vi "Bus Interface.vi"(0 "AddressSpace":refnum<class "AddressSpace.lvclass">, 1 "abort":bool, 5 "instruction":T2, 9 "input valid":bool) -> (6 "response":T1, 10 "done":bool, 14 "ready for input":bool)   [LabVIEW 2017, in "BuckBoost.lvlib" / "AddressSpace.lvclass"]
uses:
  AddressSpace.lvclass
  <instrlib>/_niInstr/Instruction Framework/v1/FPGA/Interfaces/Address Space/Address Space Instruction.ctl
  <instrlib>/_niInstr/Instruction Framework/v1/FPGA/Typedefs/Response.ctl
  AddressSpace.lvclass/AddressSpace.ctl
  <vilib>/Utility/error.llb/Clear Errors.vi
  <vilib>/rvi/Emulation/niFpgaSctlEmulationGetInTimedLoop.vi
  <vilib>/rvi/DataTransferAndStorage/Container/Common/niFpgaContainerExecOnDevCompGetState.vi
  <vilib>/rvi/Emulation/niFpgaEmulationIsFPGAContextNoSignature.vi
  <vilib>/rvi/DataTransferAndStorage/Container/Common/niFpgaContainerGetUniqueNameForEmu.vi
  <vilib>/rvi/Memory/Memory_Emulation/niFpgaMemoryEmulationCacheClearOnFirstRun.vi
  <vilib>/rvi/Memory/Memory_Emulation/nirvimemoryEmulationManagerCache_MakeExclusive.vi
  <vilib>/rvi/Memory/Memory_Emulation/niFpgaMemoryEmulationValidateCache.vi
  <vilib>/rvi/Memory/Memory_Emulation/nirvimemoryEmulationManagerCache_InsertValue.vi
  <vilib>/rvi/Memory/Memory_Emulation/nirvimemoryEmulationManagerCache_ReleaseExclusive.vi
  <vilib>/rvi/Memory/Memory_Emulation/nirvimemoryEmulationManagerCache_GetValue.vi
  <vilib>/rvi/Memory/Memory_Emulation/nirvimemoryEmulationManagerCache_SetValue.vi
  <vilib>/rvi/Emulation/niFpgaProcessEmulError.vi
  <vilib>/rvi/DataTransferAndStorage/Container/XNode/niFpgaContainer.xnode
  <vilib>/rvi/DataTransferAndStorage/Register/Emulation/niFpgaRegisterEmulationRefIn.vi
  <instrlib>/_niInstr/Instruction Framework/v1/FPGA/Typedefs/niInstr Instruction Framework v1 FPGA.lvlib
  <instrlib>/_niInstr/Instruction Framework/v1/FPGA/Interfaces/Address Space/Address Space.lvclass
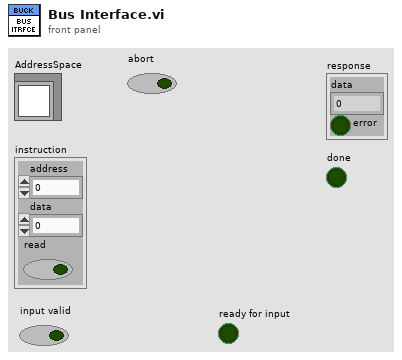
[diagram p1: front panel]
types:
  T1 = typedef "niInstr Instruction Framework v1 FPGA.lvlib/Response.ctl" = cluster{"data":u64, "error":bool}
  T2 = typedef "niInstr Instruction Framework Interfaces v1 FPGA.lvlib/Address Space.lvclass/Address Space Instruction.ctl" = cluster{"address":u32, "data":u64, "read":bool}
  T3 = cluster{"proportional gain":sgl, "integral gain":sgl}
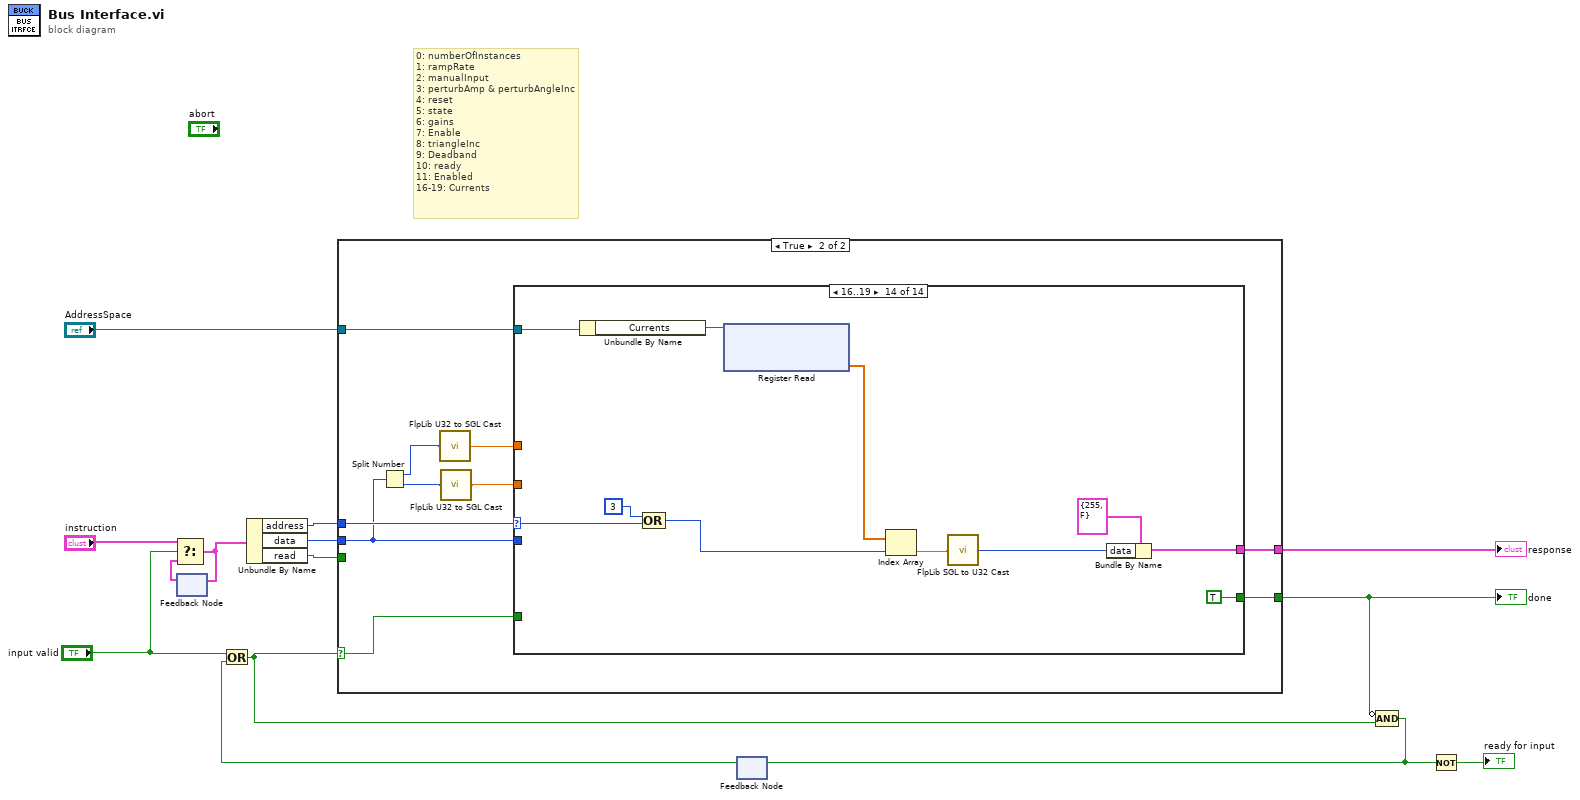
[diagram p0: block diagram]
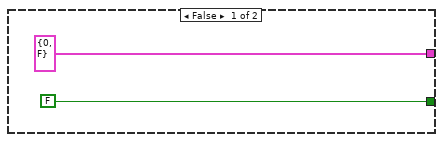
[diagram p2: hidden frame]
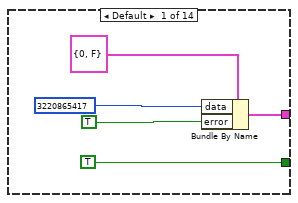
[diagram p3: hidden frame]
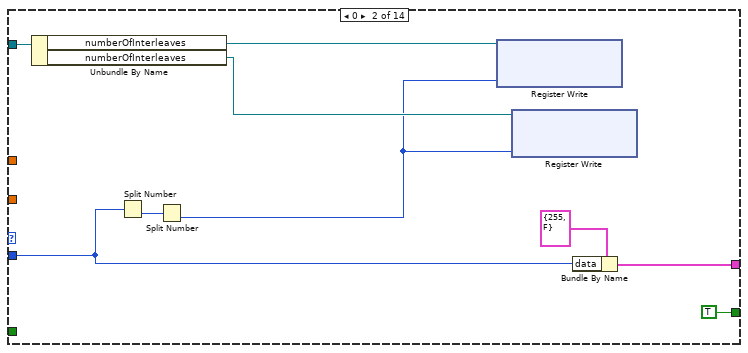
[diagram p4: hidden frame]
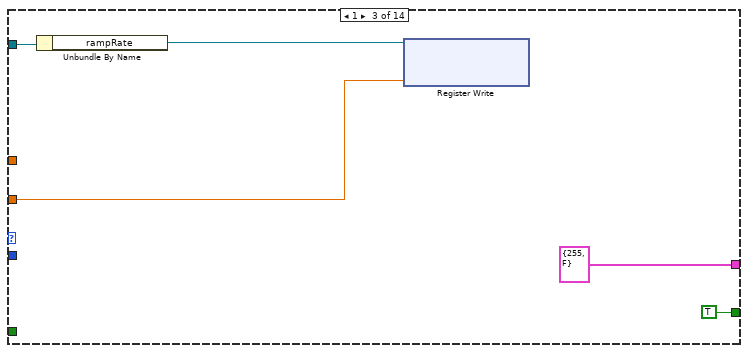
[diagram p5: hidden frame]
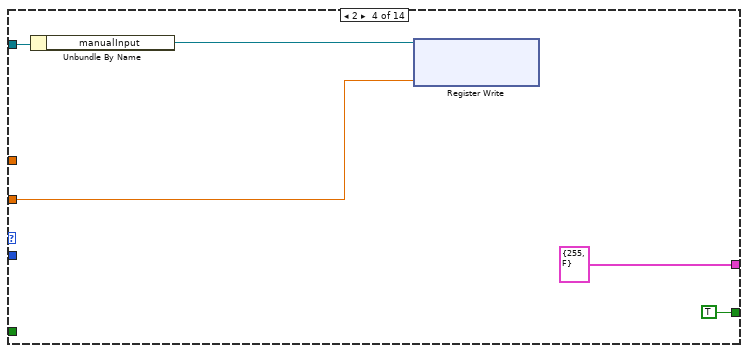
[diagram p6: hidden frame]
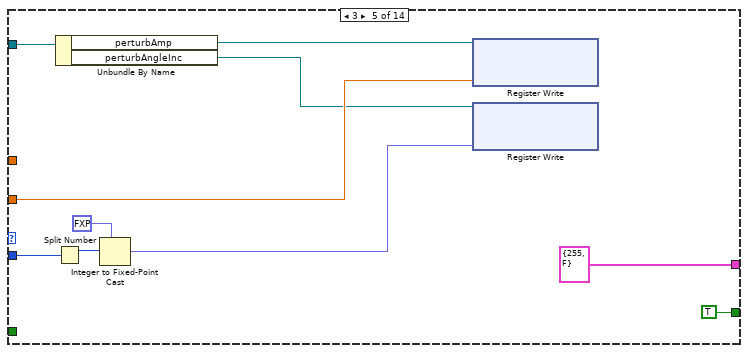
[diagram p7: hidden frame]
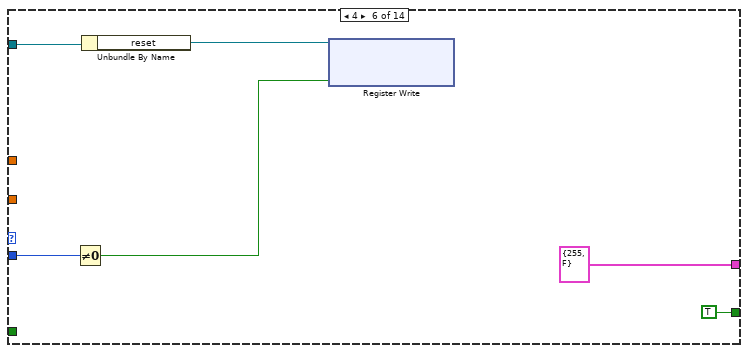
[diagram p8: hidden frame]
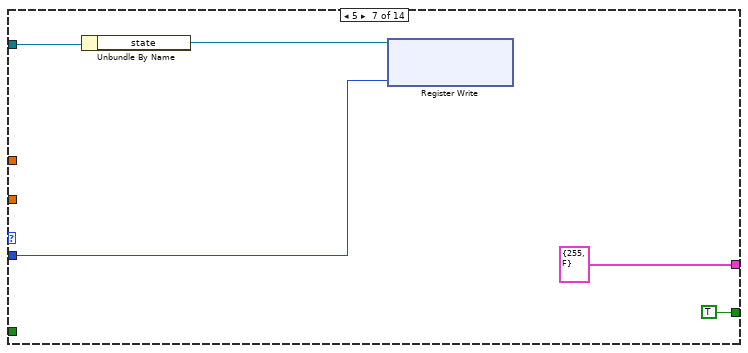
[diagram p9: hidden frame]
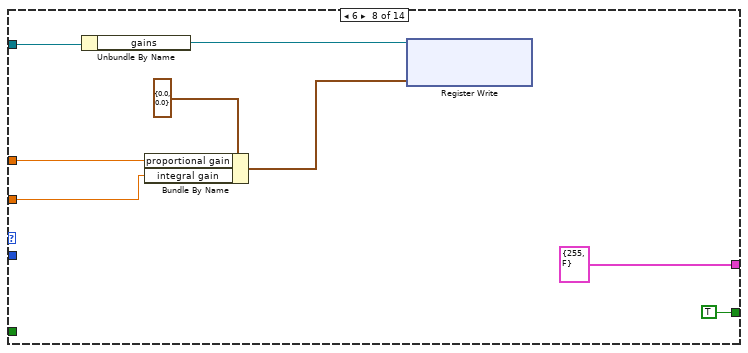
[diagram p10: hidden frame]
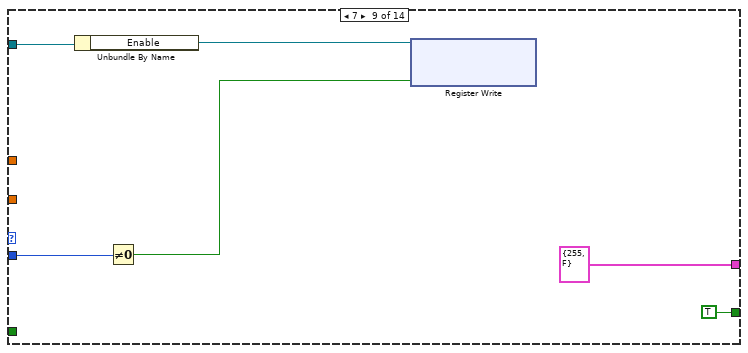
[diagram p11: hidden frame]
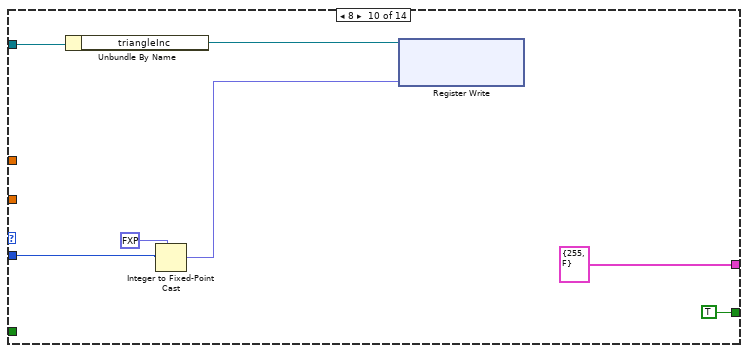
[diagram p12: hidden frame]
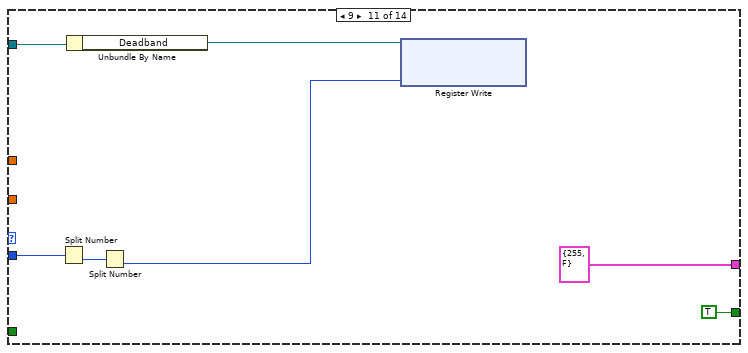
[diagram p13: hidden frame]
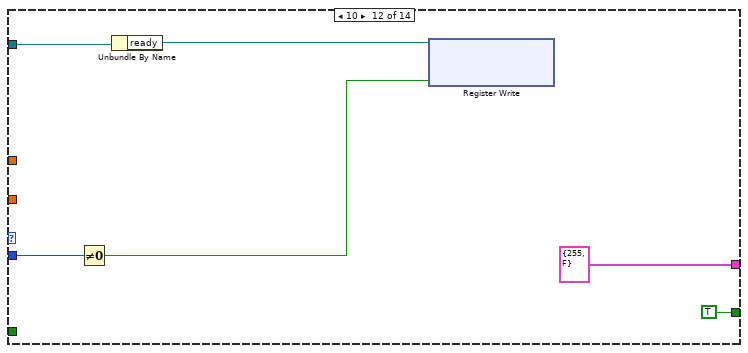
[diagram p14: hidden frame]
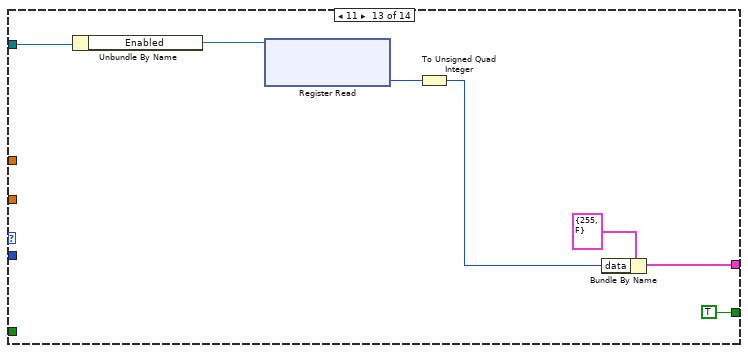
[diagram p15: hidden frame]
diagram:
  # "0: numberOfInstances\n1: rampRate\n2: manualInput\n3: perturbAmp & perturbAngleInc\n4: reset\n5: state\n6: gains\n7: Enable\n8: triangleInc\n9: Deadband\n10: ready\n11: Enabled\n16-19: Currents"
  n1 = feedback #1() -> (w14:T2)  [unwired: 1 in]
  n2 = Select(t="instruction", s="input valid", f=w14) -> (s? t:f=w13:T2)
  n3 = feedback-in #1(w13) -> ()
  n4 = Unbundle By Name(w13) -> ("address"=w10:u32, "data"=w11:u64, "read"=w12:bool)
  n5 = feedback #2() -> (w7:bool)  [unwired: 1 in]
  n6 = Or(x="input valid", y=w7) -> (x .or. y?=w8:bool)
  n7 = case shown="True" w8 {
    selector: w8 -> [_ w22]
    tunnel: w12 -> [_ _]
    tunnel: w10 -> [_ w26]
    tunnel: w11 -> [_ w21]
    tunnel: [T1 {"data"=0, "error"=FALSE} ("response") w25] -> w3
    tunnel: [FALSE ("Output Valid") w24] -> w2
    tunnel: "AddressSpace" -> [_ w23]
    frame False {
    }
    frame True {
      n8 = Split Number(x=w21) -> (hi(x)=w20:u32, lo(x)=w18:u32)
      n9 = call <userlib>:"FlpLib U32 to SGL Cast.vi"("x"=w20) -> ("y"=w19:sgl)  [unwired: 4 in]
      n10 = call <userlib>:"FlpLib U32 to SGL Cast.vi"("x"=w18) -> ("y"=w17:sgl)  [unwired: 4 in]
      n11 = case shown="16..19" w26 {
        selector: w26 -> [_ _ _ _ _ _ _ _ _ _ _ _ _ w115]
        tunnel: w21 -> [_ w36 _ _ w57 w63 w67 _ w82 w89 w96 w102 _ _]
        tunnel: [w28 w35 T1 {"data"=255, "error"=FALSE} ("response") T1 {"data"=255, "error"=FALSE} ("response") T1 {"data"=255, "error"=FALSE} ("response") T1 {"data"=255, "error"=FALSE} ("response") T1 {"data"=255, "error"=FALSE} ("response") T1 {"data"=255, "error"=FALSE} ("response") T1 {"data"=255, "error"=FALSE} ("response") T1 {"data"=255, "error"=FALSE} ("response") T1 {"data"=255, "error"=FALSE} ("response") T1 {"data"=255, "error"=FALSE} ("response") w107 w119] -> w25
        tunnel: [TRUE ("done") TRUE ("done") TRUE ("done") TRUE ("done") TRUE ("done") TRUE ("done") TRUE ("done") TRUE ("done") TRUE ("done") TRUE ("done") TRUE ("done") TRUE ("done") TRUE ("done") TRUE ("done")] -> w24
        tunnel: w23 -> [_ w40 w45 w50 w60 w66 w71 w79 w85 w92 w99 w105 w112 w123]
        tunnel: w22 -> [_ _ _ _ _ _ _ _ _ _ _ _ _ _]
        tunnel: w19 -> [_ _ _ _ _ _ _ w75 _ _ _ _ _ _]
        tunnel: w17 -> [_ _ w41 w46 w53 _ _ w74 _ _ _ _ _ _]
        frame Default {
          n12 = Bundle By Name(cluster=T1 {"data"=0, "error"=FALSE} ("response"), "data"=u64 3220865417, "error"=TRUE) -> (w28:T1)
        }
        frame 0 {
          n13 = Unbundle By Name(w40) -> ("numberOfInterleaves"=w34:refnum<k21>, "numberOfInterleaves"=w33:refnum<k21>)
          n14 = Split Number(x=w36) -> (lo(x)=w39:u32)  [unwired: 1 out]
          n15 = Split Number(x=w39) -> (lo(x)=w32:u16)  [unwired: 1 out]
          n16 = xnode ("Register Write")("Data"=w32, "Register In"=w34) -> ()  [unwired: 1 out]
          n17 = xnode ("Register Write")("Data"=w32, "Register In"=w33) -> ()  [unwired: 1 out]
          n18 = Bundle By Name(cluster=T1 {"data"=255, "error"=FALSE} ("response"), "data"=w36) -> (w35:T1)
        }
        frame 1 {
          n19 = Unbundle By Name(w45) -> ("rampRate"=w42:refnum<k21>)
          n20 = xnode ("Register Write")("Data"=w41, "Register In"=w42) -> ()  [unwired: 1 out]
        }
        frame 2 {
          n21 = Unbundle By Name(w50) -> ("manualInput"=w47:refnum<k21>)
          n22 = xnode ("Register Write")("Data"=w46, "Register In"=w47) -> ()  [unwired: 1 out]
        }
        frame 3 {
          n23 = Split Number(x=w57) -> (hi(x)=w56:u32)  [unwired: 1 out]
          n24 = Unbundle By Name(w60) -> ("perturbAmp"=w54:refnum<k21>, "perturbAngleInc"=w52:refnum<k21>)
          n25 = Integer to Fixed-Point Cast(fixed-point type=fxp<+/-,16,0> 0.0 ("Data"), integer=w56) -> (fixed-point=w51:fxp<+/-,16,0>)
          n26 = xnode ("Register Write")("Data"=w53, "Register In"=w54) -> ()  [unwired: 1 out]
          n27 = xnode ("Register Write")("Data"=w51, "Register In"=w52) -> ()  [unwired: 1 out]
        }
        frame 4 {
          n28 = Not Equal To 0?(x=w63) -> (x != 0?=w61:bool)
          n29 = Unbundle By Name(w66) -> ("reset"=w62:refnum<k21>)
          n30 = xnode ("Register Write")("Data"=w61, "Register In"=w62) -> ()  [unwired: 1 out]
        }
        frame 5 {
          n31 = Unbundle By Name(w71) -> ("state"=w68:refnum<k21>)
          n32 = xnode ("Register Write")("Data"=w67, "Register In"=w68) -> ()  [unwired: 1 out]
        }
        frame 6 {
          n33 = Unbundle By Name(w79) -> ("gains"=w73:refnum<k21>)
          n34 = Bundle By Name(cluster=T3 {"proportional gain"=0.0, "integral gain"=0.0} ("Data"), "proportional gain"=w75, "integral gain"=w74) -> (w72:T3)
          n35 = xnode ("Register Write")("Data"=w72, "Register In"=w73) -> ()  [unwired: 1 out]
        }
        frame 7 {
          n36 = Unbundle By Name(w85) -> ("Enable"=w81:refnum<k21>)
          n37 = Not Equal To 0?(x=w82) -> (x != 0?=w80:bool)
          n38 = xnode ("Register Write")("Data"=w80, "Register In"=w81) -> ()  [unwired: 1 out]
        }
        frame 8 {
          n39 = Unbundle By Name(w92) -> ("triangleInc"=w87:refnum<k21>)
          n40 = Integer to Fixed-Point Cast(fixed-point type=fxp<+,18,0> 0.0 ("Data"), integer=w89) -> (fixed-point=w86:fxp<+,18,0>)
          n41 = xnode ("Register Write")("Data"=w86, "Register In"=w87) -> ()  [unwired: 1 out]
        }
        frame 9 {
          n42 = Split Number(x=w96) -> (lo(x)=w95:u32)  [unwired: 1 out]
          n43 = Unbundle By Name(w99) -> ("Deadband"=w94:refnum<k21>)
          n44 = Split Number(x=w95) -> (lo(x)=w93:u16)  [unwired: 1 out]
          n45 = xnode ("Register Write")("Data"=w93, "Register In"=w94) -> ()  [unwired: 1 out]
        }
        frame 10 {
          n46 = Not Equal To 0?(x=w102) -> (x != 0?=w100:bool)
          n47 = Unbundle By Name(w105) -> ("ready"=w101:refnum<k21>)
          n48 = xnode ("Register Write")("Data"=w100, "Register In"=w101) -> ()  [unwired: 1 out]
        }
        frame 11 {
          n49 = Unbundle By Name(w112) -> ("Enabled"=w110:refnum<k21>)
          n50 = xnode ("Register Read")("Register In"=w110) -> ("Data"=w106:u8)  [unwired: 1 out]
          n51 = To Unsigned Quad Integer(1:w106) -> (0:w108:u64)
          n52 = Bundle By Name(cluster=T1 {"data"=255, "error"=FALSE} ("response"), "data"=w108) -> (w107:T1)
        }
        frame 16..19 {
          n53 = Unbundle By Name(w123) -> ("Currents"=w121:refnum<k21>)
          n54 = Compound Arithmetic op=OR(u32 3 ("value"), w115) -> (w113:u32)
          n55 = xnode ("Register Read")("Register In"=w121) -> ("Data"=w118:sgl[])  [unwired: 1 out]
          n56 = Index Array(array=w118, index=w113) -> (element=w117:sgl)
          n57 = call <userlib>:"FlpLib SGL to U32 Cast.vi"("x"=w117) -> ("y"=w116:u32)  [unwired: 4 in]
          n58 = Bundle By Name(cluster=T1 {"data"=255, "error"=FALSE} ("response"), "data"=w116) -> (w119:T1)
        }
      }
    }
  }
  "done" <- w2
  "response" <- w3
  n59 = Compound Arithmetic op=AND(invert w2, w8) -> (w9:bool)
  n60 = feedback-in #2(w9) -> ()
  n61 = Not(x=w9) -> (.not. x?=→"ready for input":bool)
